vi "denois2.vi"() -> ()   [LabVIEW 2019]
uses:
  <vilib>/measure/mamon.llb/Trigger Detection for 1 Channel.vi
  <vilib>/measure/NI_MAPro.lvlib
panel:
  out "Waveform Chart 4":waveform(dbl)(graph)
  out "x+1":dbl
  out "Waveform Chart 3":waveform(dbl)(graph)
  out "trigger detected?":bool
  in  "stop":bool
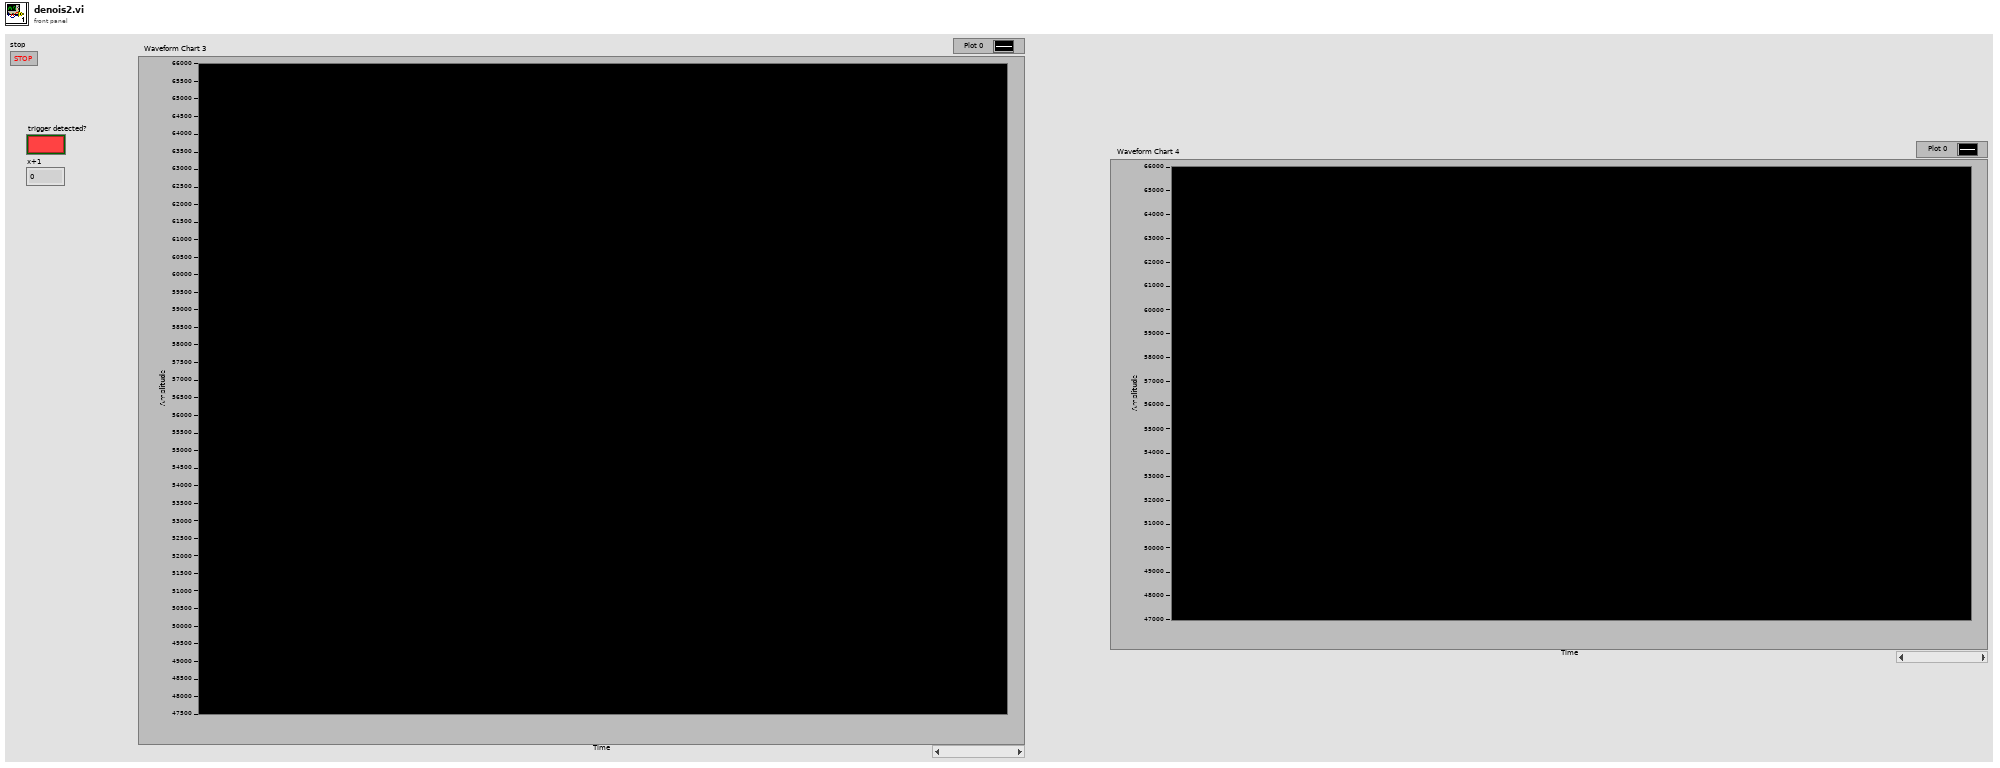
[diagram p1: front panel]
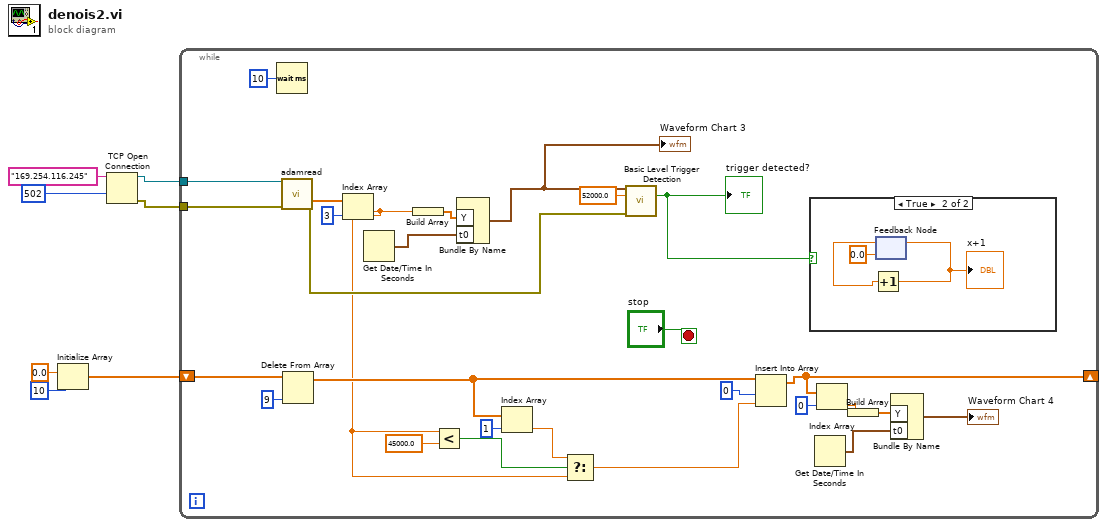
[diagram p0: block diagram]
diagram:
  n1 = Initialize Array(0.0 ("element"), 10 ("dimension size")) -> (w1:dbl[])
  n2 = TCP Open Connection(address="169.254.116.245", remote port or service name=u16 502) -> (connection ID=w5:refnum<k5>, error out=w4:errorcluster)  [unwired: 3 in]
  n3 = while {
    tunnel: w5 -> [w34]
    tunnel: w4 -> [w33]
    shift-right: [w11] -> _
    shift-left: w1 -> [w23]
    stop <- "stop" stop-if-true
    n4 = Wait (ms)(milliseconds to wait=u32 10) -> ()  [unwired: 1 out]
    n5 = call "adamread.vi"("TCP Connection Refnum in"=w34, "error in (no error)"=w33) -> ("Slave Input Registers 2"=w32:dbl[], "error out 2"=w27:errorcluster)  [unwired: 11 in, 1 out]
    n6 = Delete From Array(array=w23, index=9) -> (array with subset deleted=w18:dbl[])  [unwired: 1 in, 1 out]
    n7 = Index Array(array=w32, index=3) -> (element=w15:dbl)
    n8 = Get Date/Time In Seconds() -> (seconds since 1Jan1904=w29:timestamp)
    n9 = Build Array(w15) -> (w30:dbl[])
    n10 = Less?(x=w15, y=45000.0) -> (x < y?=w19:bool)
    n11 = Bundle By Name("Y"=w30, "t0"=w29) -> (w26:waveform(dbl))  [unwired: 1 in]
    "Waveform Chart 3" <- w26
    n12 = Index Array(array=w18, index=1) -> (element=w16:dbl)
    n13 = Select(t=w16, s=w19, f=w15) -> (s? t:f=w14:dbl)
    n14 = call-poly <vilib>:"Basic Level Trigger Detection.vi"("signal in"=w26, "level"=52000.0, "error in (no error)"=w27) -> ("trigger detected?"=w24:bool)  [unwired: 10 in, 2 out]
    "trigger detected?" <- w24
    n15 = Insert Into Array(array=w18, index=0, new element=w14) -> (w11:dbl[])
    n16 = case shown="True" w24 {
      frame False {
      }
      frame True {
        n17 = feedback #1(0.0) -> (w37:dbl)
        n18 = Increment(x=w37) -> (x+1=w38:dbl)
        "x+1" <- w38
        n19 = feedback-in #1(w38) -> ()
      }
    }
    n20 = Get Date/Time In Seconds() -> (seconds since 1Jan1904=w13:timestamp)
    n21 = Index Array(array=w11, index=0) -> (element=w9:dbl)
    n22 = Build Array(w9) -> (w8:dbl[])
    n23 = Bundle By Name("Y"=w8, "t0"=w13) -> (→"Waveform Chart 4":waveform(dbl))  [unwired: 1 in]
  }
